vi "getU8Array.vi"(6 "length":i32, 7 "offset":i32, 8 "String":string) -> (3 "array":u8[](array[numeric]))   [LabVIEW 2013]
doc: "Get an array of U8 with length elements from string at offset"
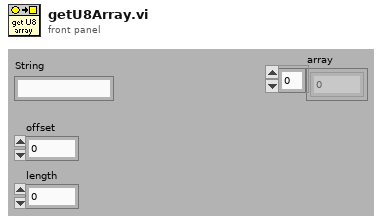
[diagram p1: front panel]
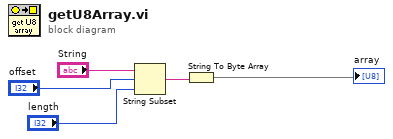
[diagram p0: block diagram]
diagram:
  n1 = String Subset(string="String", offset (0)="offset", length (rest)="length") -> (substring=w3:string)
  n2 = String To Byte Array(string=w3) -> (unsigned byte array=→"array":u8[])
